vi "ReadFileDialog.vi"(6 "File Text":string, 8 "error in (no error)":errorcluster, 9 "File name":string, 10 "Console in":string, 11 "Python in":T1) -> (0 "error out":errorcluster, 2 "Console":string)   [LabVIEW 2022 SP3]
uses:
  PythonCtrl.ctl
  Processors.ctl
  <vilib>/Utility/error.llb/Trim Whitespace One-Sided.vi
  Comm_Global.vi
panel:
  out "diff":i16
  out "File received":string
  out "File Sent":string
  in  "Done":bool
  in  "Abort":bool
  out "Python out":T1
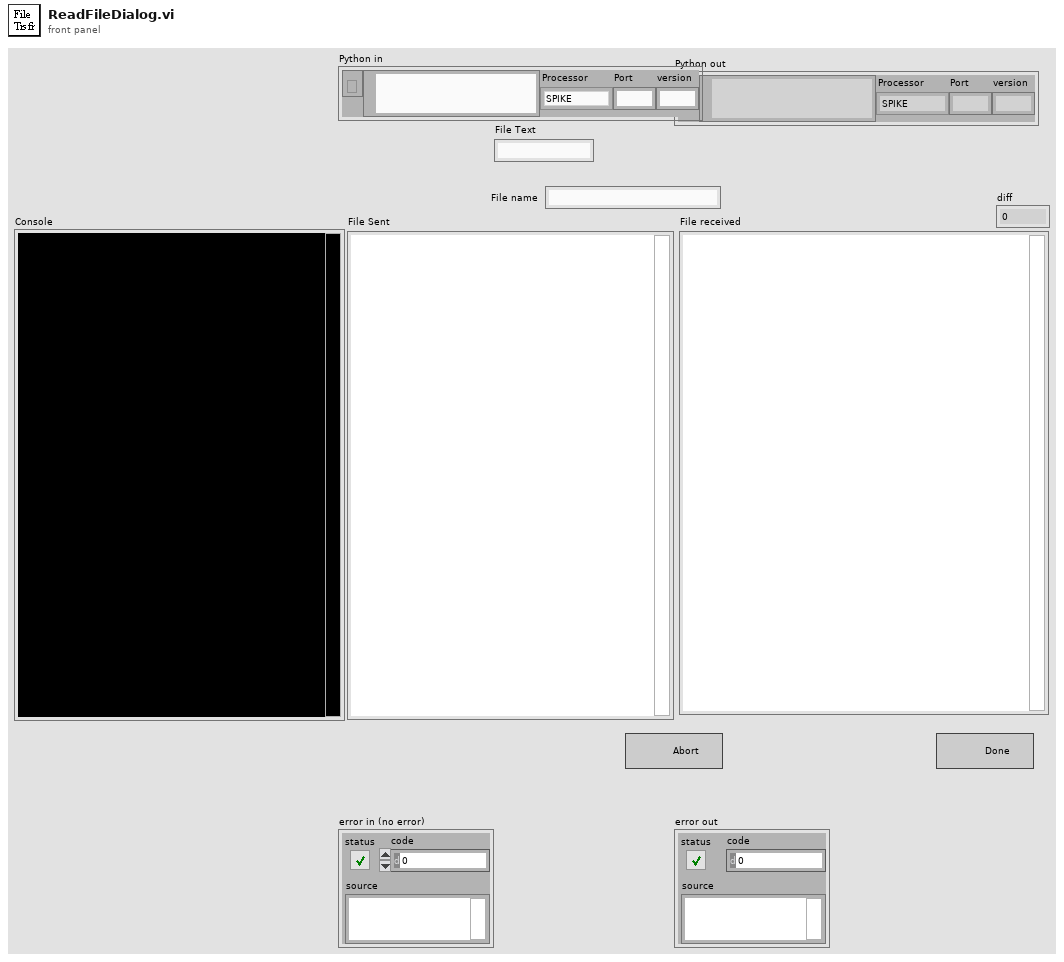
[diagram p1: front panel]
types:
  T1 = typedef "PythonCtrl.ctl" = cluster{"session":refnum<k35>, "PyPath":path, "Processor":T2, "Port":string, "version":string}
  T2 = typedef "Processors.ctl" = enum16{"SPIKE", "Pi", "Pi_ssh", "OpenMV", "Dunio"}
  T3 = enum32{"Invalid", "Standard", "Closed", "Hidden", "Minimized", "Maximized"}
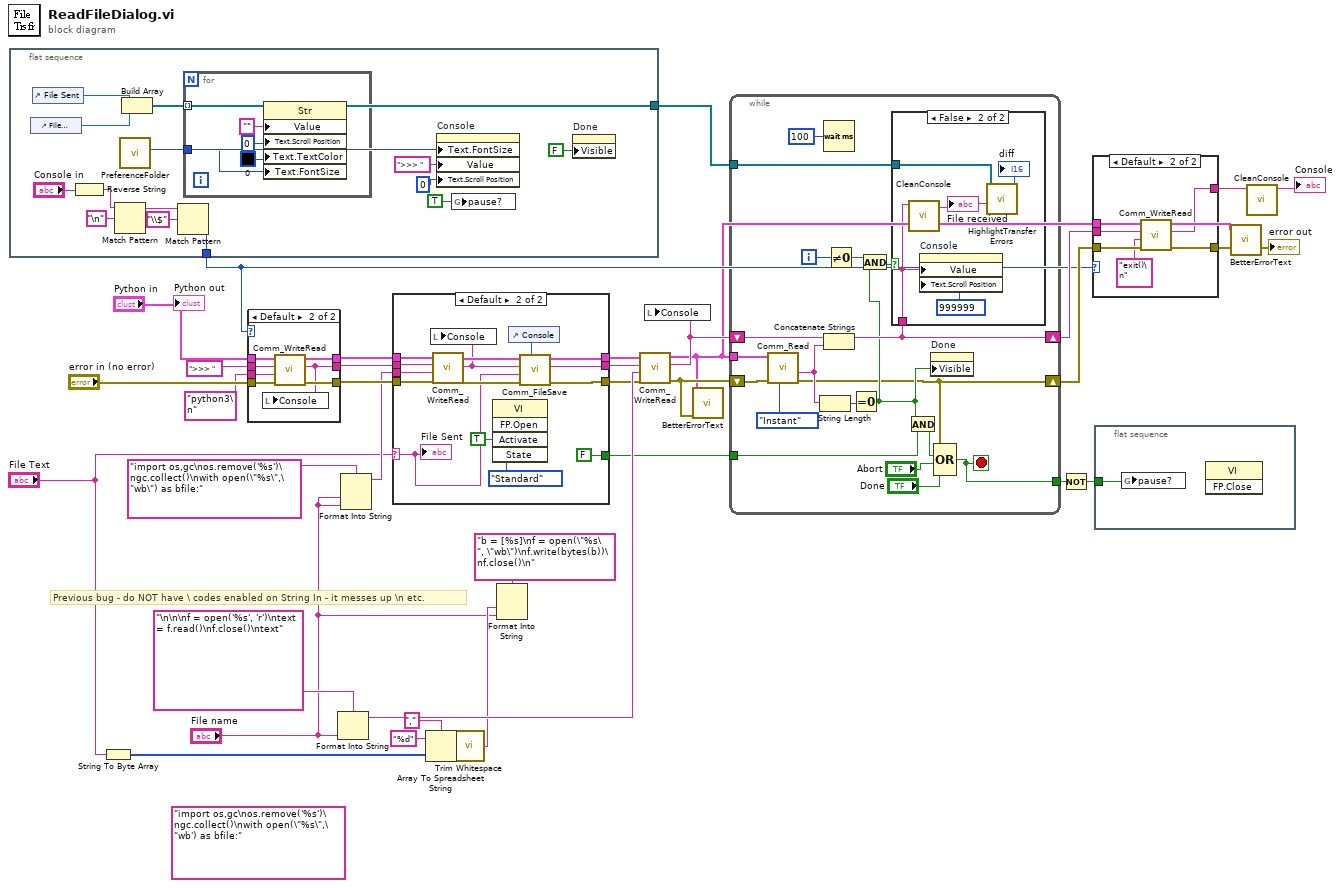
[diagram p0: block diagram]
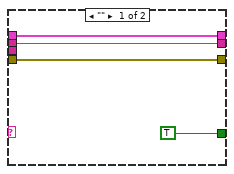
[diagram p4: hidden frame]
diagram:
  (unwired) "import os,gc\nos.remove('%s')\ngc.collect()\nwith open(\"%s\",\"wb') as bfile:" ("function name")
  # "Previous bug - do NOT have \\ codes enabled on String In - it messes up \\n etc."
  n1 = flat-sequence {
    tunnel: [w47] -> w18
    tunnel: [w37] -> w12
    frame #0 {
      n2 = control-ref of="File received"() -> (w48:refnum<vi>)
      n3 = control-ref of="File Sent"() -> (w49:refnum<vi>)
      n4 = Reverse String(1:"Console in") -> (0:w41:string)
      n5 = Match Pattern(string=w41, regular expression="\n") -> (before substring=w42:string)  [unwired: 1 in, 3 out]
      n6 = call "PreferenceFolder.vi"() -> ("FontSize"=w36:u8)  [unwired: 5 in, 6 out]
      n7 = Build Array(w49, w48) -> (w47:refnum<vi>[])
      n8 = Match Pattern(string=w42, regular expression="\\$") -> (offset past match=w37:i32)  [unwired: 1 in, 3 out]
      n9 = for {
        tunnel: w47 -> [w54] mode=indexing
        tunnel: w36 -> [w50]
        n10 = property on="Property Node" class="Str"(reference=w54, "Value"="", "Text.Scroll Position"=u32 0, "Text.TextColor"=u32 0 ("Text.Text Colors:Text Color"), "Text.FontSize"=w50) -> ()  [unwired: 1 in, 2 out]
      }
      n11 = property on="Console" class="Str"("Text.FontSize"=w36, "Value"=">>> " ("Console"), "Text.Scroll Position"=u32 0) -> ()  [unwired: 2 in, 2 out]
      n12 = global write "Comm_Global.vi" "pause?"(TRUE ("pause?")) -> ()
      n13 = property on="Done" class="Bool"("Visible"=FALSE) -> ()  [unwired: 2 in, 2 out]
    }
  }
  n14 = String To Byte Array(string="File Text") -> (unsigned byte array=w6:u8[])
  n15 = case shown="Default" w12 {
    tunnel: [w55 w64] -> w27
    tunnel: [w56 w58] -> w26
    tunnel: [w57 w63] -> w25
    tunnel: "Python in" -> [w57 w62]
    tunnel: ">>> " ("Text to write") -> [w56 w61]
    tunnel: "error in (no error)" -> [w55 w60]
    tunnel: "python3\n" ("regular expression") -> [_ w59]
    frame -1 {
    }
    frame Default {
      n16 = call "Comm_WriteRead.vi"("error in (no error)"=w60, "Code"=w59, "Console In"=w61, "Python"=w62) -> ("error out"=w64:errorcluster, "Console"=w58:string, "Python"=w63:T1)  [unwired: 5 in]
      n17 = local write "Console"(w58) -> ()
    }
  }
  n18 = Format Into String(format string="\n\n\nf = open('%s', 'r')\ntext = f.read()\nf.close()\ntext" ("function name"), "File name") -> (resulting string=w35:string)  [unwired: 2 in, 1 out]
  n19 = Format Into String(format string="import os,gc\nos.remove('%s')\ngc.collect()\nwith open(\"%s\",\"wb\") as bfile:" ("function name"), "File name", "File name") -> (resulting string=w13:string)  [unwired: 2 in, 1 out]
  n20 = case shown="Default" "File Text" {
    selector: "File Text" -> [_ w69]
    tunnel: [w66 w74] -> w32
    tunnel: [w67 w72] -> w31
    tunnel: [w68 w73] -> w30
    tunnel: w25 -> [w68 w81]
    tunnel: w26 -> [w67 w82]
    tunnel: w27 -> [w66 w83]
    tunnel: [TRUE FALSE] -> w17
    tunnel: w13 -> [_ w79]
    frame "" {
    }
    frame Default {
      n21 = call "Comm_WriteRead.vi"("error in (no error)"=w83, "Code"=w79, "Console In"=w82, "Python"=w81) -> ("error out"=w75:errorcluster, "Console"=w71:string, "Python"=w76:T1)  [unwired: 5 in]
      n22 = local write "Console"(w71) -> ()
      n23 = invoke class="VI" method="FP.Open"("Activate"=TRUE ("Activate?"), "State"=T3."Standard") -> ()  [unwired: 3 in, 5 out]
      n24 = control-ref of="Console"() -> (w70:refnum<vi>)
      n25 = call "Comm_FileSave.vi"("Console"=w70, "error in (no error)"=w75, "Code"=w69, "Console In"=w71, "Python"=w76) -> ("error out"=w74:errorcluster, "Console"=w72:string, "Python"=w73:T1)  [unwired: 4 in]
      "File Sent" <- w69
    }
  }
  n26 = Array To Spreadsheet String(delimiter (Tab)=",", array=w6, 3:"%d" ("format string")) -> (spreadsheet string=w3:string)
  n27 = call <vilib>:"Trim Whitespace.vi"("string"=w3) -> ("trimmed string"=w2:string)  [unwired: 1 in]
  n28 = Format Into String(format string="b = [%s]\nf = open(\"%s\", \"wb\")\nf.write(bytes(b))\nf.close()\n" ("function name"), w2, "File name") -> ()  [unwired: 2 in, 2 out]
  n29 = call "Comm_WriteRead.vi"("error in (no error)"=w32, "Code"=w35, "Console In"=w31, "Python"=w30) -> ("error out"=w9:errorcluster, "Console"=w29:string, "Python"=w8:T1)  [unwired: 5 in]
  n30 = local write "Console"(w29) -> ()
  n31 = call "BetterErrorText.vi"("error in (no error)"=w9, "Python"=w8) -> ()  [unwired: 8 in, 2 out]
  n32 = while {
    shift-right: [w97] -> w19
    shift-left: w29 -> [w100]
    tunnel: w8 -> [w98]
    shift-right: [w84] -> w20
    shift-left: w9 -> [w101]
    tunnel: [w93] -> w28
    tunnel: w18 -> [w92]
    tunnel: w17 -> [w91]
    i -> [w87]
    stop <- w93 stop-if-true
    n33 = call "Comm_Read.vi"("Task"=enum16{"Instant", "All"}."Instant", "error in (no error)"=w101, "Python"=w98) -> ("error out"=w84:errorcluster, "Text read"=w99:string)  [unwired: 7 in]
    n34 = String Length(string=w99) -> (length=w94:i32)
    n35 = Wait (ms)(milliseconds to wait=u32 100) -> ()  [unwired: 1 out]
    n36 = Concatenate Strings(w100, w99) -> (w97:string)
    n37 = Not Equal To 0?(x=w87) -> (x != 0?=w88:bool)
    n38 = Equal To 0?(x=w94) -> (x = 0?=w86:bool)
    n39 = And(x=w88, y=w86) -> (x .and. y?=w85:bool)
    n40 = case shown="False" w85 {
      tunnel: w97 -> [_ w106]
      tunnel: w92 -> [_ w105]
      frame True {
      }
      frame False {
        n41 = call "CleanConsole.vi"("Console in"=w106) -> ("Console out"=w103:string)  [unwired: 10 in]
        "File received" <- w103
        n42 = property on="Console" class="Str"("Value"=w106, "Text.Scroll Position"=u32 999999) -> ()  [unwired: 2 in, 2 out]
        n43 = call "HighlightTransferErrors.vi"("File received"=w103, "Sent/Recieved"=w105) -> ("diff"=→"diff":i16)  [unwired: 9 in]
      }
    }
    n44 = And(x=w86, y=w91) -> (x .and. y?=w90:bool)
    n45 = property on="Done" class="Bool"("Visible"=w86) -> ()  [unwired: 2 in, 2 out]
    n46 = Compound Arithmetic op=OR(w84, w90, "Abort", "Done") -> (w93:bool)
  }
  n47 = Not(x=w28) -> (.not. x?=w11:bool)
  n48 = case shown="Default" w12 {
    tunnel: [w109 w115] -> w10
    tunnel: w8 -> [_ w114]
    tunnel: w19 -> [w108 w113]
    tunnel: w20 -> [w109 w112]
    tunnel: [w108 w110] -> w16
    frame -1 {
    }
    frame Default {
      n49 = call "Comm_WriteRead.vi"("error in (no error)"=w112, "Code"="exit()\n" ("regular expression"), "Console In"=w113, "Python"=w114) -> ("error out"=w115:errorcluster, "Console"=w110:string)  [unwired: 5 in, 1 out]
    }
  }
  "error out" <- w10
  n50 = flat-sequence {
    tunnel: w11 -> [w116]
    frame #0 {
      n51 = global write "Comm_Global.vi" "pause?"(w116) -> ()
      n52 = invoke class="VI" method="FP.Close"() -> ()  [unwired: 3 in, 3 out]
    }
  }
  n53 = call "BetterErrorText.vi"("error in (no error)"=w10, "Python"=w8) -> ()  [unwired: 8 in, 2 out]
  n54 = call "CleanConsole.vi"("Console in"=w16) -> ("Console out"=→"Console":string)  [unwired: 10 in]
  "Python out" <- "Python in"
